vi "ConvertFromAssociationType.vi"(0 "RelationType":T1 items=["Depenency", "Inheritance", "Interface Implementation", "Association", "Aggregation", "Composite Aggregation"], 2 "Bi sirectional":bool) -> (14 "lineStyle":T3, 15 "EndArrowHead":T2, 16 "StartArrowHead":T2)   [LabVIEW 2012, in "ClassRelationshipEdge.lvclass"]
uses:
  <resource>/Framework/Providers/Open_GDS/UML/ClassRelationshipEdge_class/ClassRelationshipEdge.lvclass
  <resource>/Framework/Providers/Open_GDS/UML/ArrowHead_class/ArrowHeadType.ctl
  <resource>/Framework/Providers/Open_GDS/UML/LineStyle_class/LineStyleType.ctl
  <resource>/Framework/Providers/Open_GDS/UML/ClassRelationshipEdge_class/private/AssociationType.ctl
  <resource>/Framework/Providers/Open_GDS/UML/Graphics_class/StrokeType.ctl
  <resource>/Framework/Providers/Open_GDS/UML/ArrowHead_class/ArrowHead.lvclass
  <resource>/Framework/Providers/Open_GDS/UML/Graphics_class/Graphics.lvclass
  <resource>/Framework/Providers/Open_GDS/UML/LineStyle_class/LineStyle.lvclass
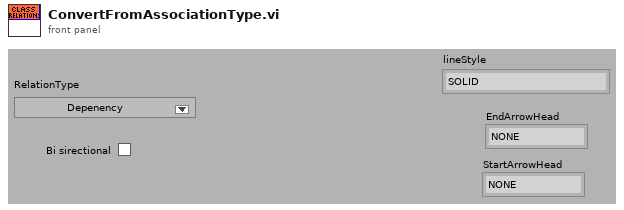
[diagram p1: front panel]
types:
  T1 = typedef "ClassRelationshipEdge.lvclass/AssociationType.ctl" = u16
  T2 = typedef "ArrowHead.lvclass/ArrowHeadType.ctl" = enum16{"NONE", "TRIANGLE", "BLACK_TRIANGLE", "V", "HALF_V", "DIAMOND", "BLACK_DIAMOND"}
  T3 = typedef "LineStyle.lvclass/LineStyleType.ctl" = enum16{"SOLID", "DOTTED"}
  T4 = typedef "Graphics.lvclass/StrokeType.ctl" = enum16{"USE_DEFAULT", "SOLID", "DOTTED"}
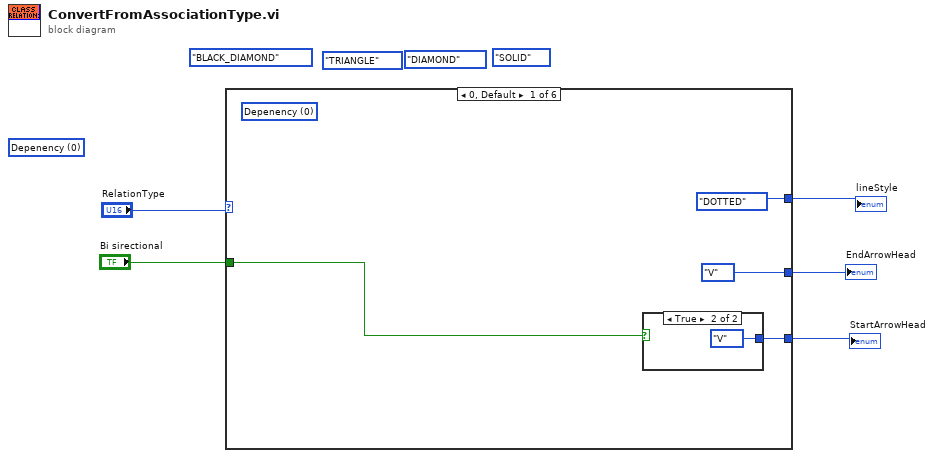
[diagram p0: block diagram]
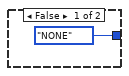
[diagram p2: hidden frame]
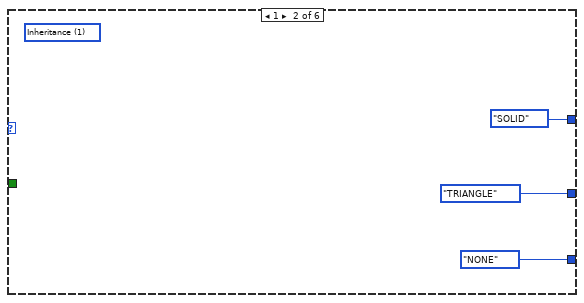
[diagram p3: hidden frame]
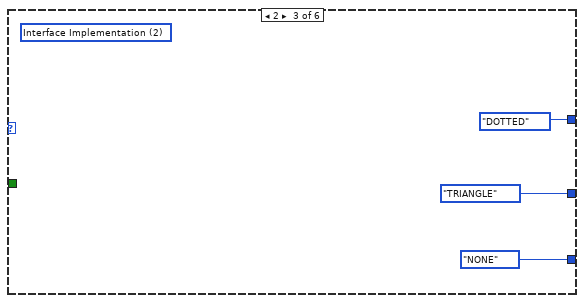
[diagram p4: hidden frame]
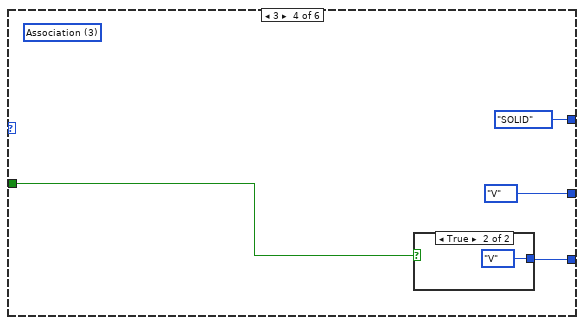
[diagram p5: hidden frame]
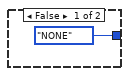
[diagram p6: hidden frame]
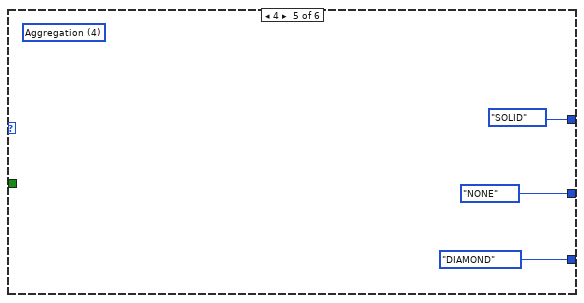
[diagram p7: hidden frame]
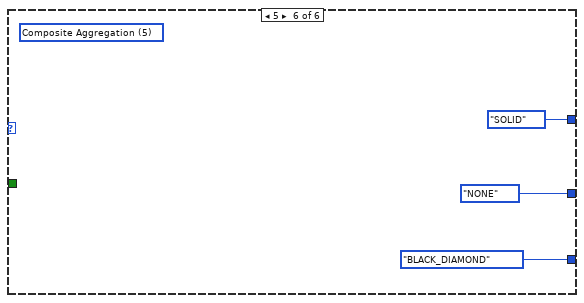
[diagram p8: hidden frame]
diagram:
  (unwired) ArrowHeadType."BLACK_DIAMOND" ("y")
  (unwired) StrokeType."SOLID" ("y")
  (unwired) ArrowHeadType."DIAMOND" ("y")
  (unwired) ArrowHeadType."TRIANGLE" ("y")
  (unwired) T1 0 items=["Depenency", "Inheritance", "Interface Implementation", "Association", "Aggregation", "Composite Aggregation"] ("RelationType")
  n1 = case shown="0, Default" "RelationType" {
    tunnel: [LineStyleType."DOTTED" ("lineStyle") LineStyleType."SOLID" ("lineStyle") LineStyleType."DOTTED" ("lineStyle") LineStyleType."SOLID" ("lineStyle") LineStyleType."SOLID" ("lineStyle") LineStyleType."SOLID" ("lineStyle")] -> w1
    tunnel: [ArrowHeadType."V" ("y") ArrowHeadType."TRIANGLE" ("y") ArrowHeadType."TRIANGLE" ("y") ArrowHeadType."V" ("y") ArrowHeadType."NONE" ("y") ArrowHeadType."NONE" ("y")] -> w4
    tunnel: [w8 ArrowHeadType."NONE" ("y") ArrowHeadType."NONE" ("y") w20 ArrowHeadType."DIAMOND" ("y") ArrowHeadType."BLACK_DIAMOND" ("y")] -> w3
    tunnel: "Bi sirectional" -> [w7 _ _ w19 _ _]
    frame 0, Default {
      (unwired) T1 0 items=["Depenency", "Inheritance", "Interface Implementation", "Association", "Aggregation", "Composite Aggregation"] ("RelationType")
      n2 = case shown="True" w7 {
        tunnel: [ArrowHeadType."NONE" ("y") ArrowHeadType."V" ("y")] -> w8
        frame False {
        }
        frame True {
        }
      }
    }
    frame 1 {
      (unwired) T1 1 items=["Depenency", "Inheritance", "Interface Implementation", "Association", "Aggregation", "Composite Aggregation"] ("RelationType")
    }
    frame 2 {
      (unwired) T1 2 items=["Depenency", "Inheritance", "Interface Implementation", "Association", "Aggregation", "Composite Aggregation"] ("RelationType")
    }
    frame 3 {
      (unwired) T1 3 items=["Depenency", "Inheritance", "Interface Implementation", "Association", "Aggregation", "Composite Aggregation"] ("RelationType")
      n3 = case shown="True" w19 {
        tunnel: [ArrowHeadType."NONE" ("y") ArrowHeadType."V" ("y")] -> w20
        frame False {
        }
        frame True {
        }
      }
    }
    frame 4 {
      (unwired) T1 4 items=["Depenency", "Inheritance", "Interface Implementation", "Association", "Aggregation", "Composite Aggregation"] ("RelationType")
    }
    frame 5 {
      (unwired) T1 5 items=["Depenency", "Inheritance", "Interface Implementation", "Association", "Aggregation", "Composite Aggregation"] ("RelationType")
    }
  }
  "EndArrowHead" <- w4
  "lineStyle" <- w1
  "StartArrowHead" <- w3
